vi "Destroy.vi"(8 "error in (no error)":errorcluster, 11 "Progress In":refnum<class "Progressbar.lvclass">) -> (0 "error out":errorcluster, 3 "Progress Out":refnum<class "Progressbar.lvclass">)   [LabVIEW 2017, in "Front Panel Publisher.lvlib" / "Progressbar.lvclass"]
uses:
  Progressbar.lvclass
  Control_class/Control.lvclass
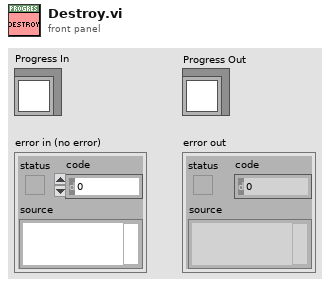
[diagram p1: front panel]
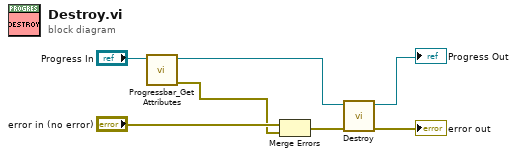
[diagram p0: block diagram]
diagram:
  n1 = call "Progressbar_Get Attributes.vi"("Progress In"="Progress In") -> ("error out"=w1:errorcluster, "Progress Out"=w5:refnum<class "Progressbar.lvclass">)  [unwired: 8 in, 1 out]
  n2 = Merge Errors("error in (no error)", w1) -> (w4:errorcluster)
  n3 = call-parent "Destroy.vi"("error in (no error)"=w4, "Control In"=w5) -> ("error out"=→"error out":errorcluster, "Control Out"=→"Progress Out":refnum<class "Progressbar.lvclass">)  [unwired: 8 in]
